vi "Write Instrument Name.vi"(8 "error in (no error)":errorcluster, 10 "Instrument Name":string, 11 "Actor_Autotest in":refnum<class "Actor_Autotest.lvclass">) -> (0 "error out":errorcluster, 3 "Actor_Autotest out":refnum<class "Actor_Autotest.lvclass">)   [LabVIEW 2020, in "Library Core.lvlib" / "Actor_Autotest.lvlib" / "Actor_Autotest.lvclass"]
uses:
  Actor_Autotest.lvclass
  Actor_Autotest.lvclass/Actor_Autotest.ctl
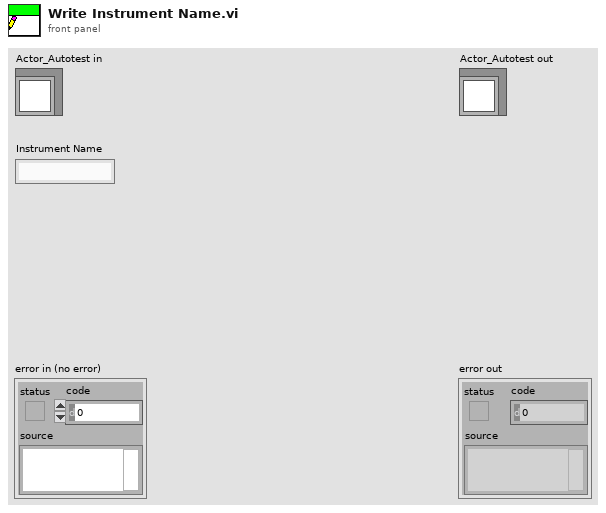
[diagram p1: front panel]
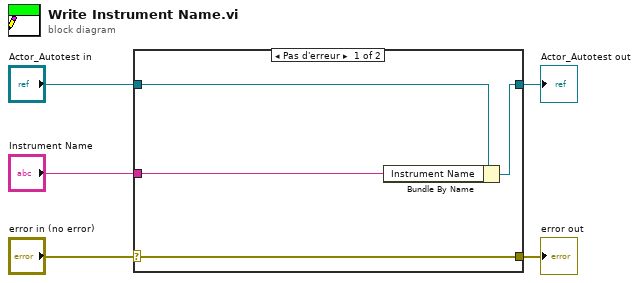
[diagram p0: block diagram]
diagram:
  n1 = case shown="Pas d'erreur" "error in (no error)" {
    selector: "error in (no error)" -> [w9 w10]
    tunnel: [w9 w10] -> w4
    tunnel: [w7 w11] -> w2
    tunnel: "Actor_Autotest in" -> [w8 w11]
    tunnel: "Instrument Name" -> [w6 _]
    frame No Error {
      n2 = Bundle By Name(cluster=w8, "Instrument Name"=w6) -> (w7:refnum<class "Actor_Autotest.lvclass">)
    }
    frame Error {
    }
  }
  "error out" <- w4
  "Actor_Autotest out" <- w2
